vi "Filter Meta.vi"(8 "error in (no error)":errorcluster, 10 "Element In":refnum<class "Config Element.lvclass">, 11 "Overlay Filter in":refnum<class "Overlay Filter.lvclass">) -> (0 "error out":errorcluster, 1 "Filtered Meta":T1[](array[typedef]), 2 "Element":refnum<class "Config Element.lvclass">, 3 "Overlay Filter out":refnum<class "Overlay Filter.lvclass">)   [LabVIEW 2020, in "CDM-Config.lvlib" / "Overlay Filter.lvclass"]
uses:
  Overlay Filter.lvclass
  Config Element/Config Element.lvclass
  Meta Data.ctl
  Overlay Filter.lvclass/Overlay Filter.ctl
  CDM-Config.lvlib
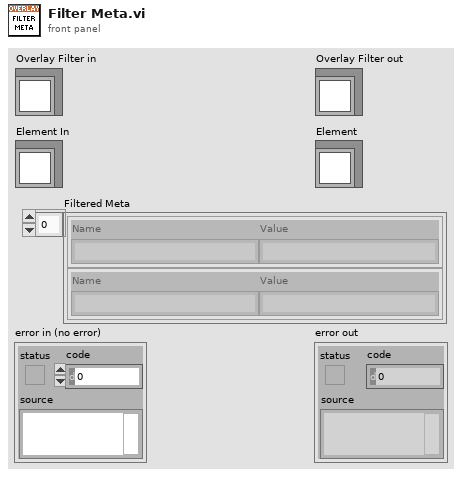
[diagram p1: front panel]
types:
  T1 = typedef "CDM-Config.lvlib/Meta Data.ctl" = cluster{"Name":string, "Value":string}
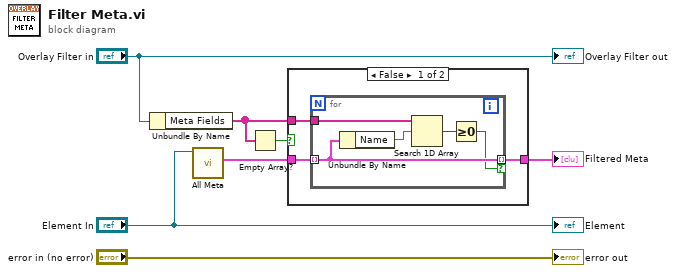
[diagram p0: block diagram]
diagram:
  n1 = Unbundle By Name("Overlay Filter in") -> ("Meta Fields"=w2:string[])
  n2 = call "All Meta.vi"("Config Element In"="Element In") -> ("Meta Data"=w5:T1[])  [unwired: 8 in, 2 out]
  n3 = Empty Array?(array=w2) -> (empty?=w1:bool)
  n4 = case shown="False" w1 {
    tunnel: w5 -> [w10 w16]
    tunnel: [w9 w16] -> w3
    tunnel: w2 -> [w8 _]
    frame False {
      n5 = for {
        tunnel: w8 -> [w15]
        tunnel: w10 -> [w14] mode=indexing
        tunnel: [w14] -> w9 mode=indexing if=w11
        n6 = Unbundle By Name(w14) -> ("Name"=w13:string)
        n7 = Search 1D Array(1D array=w15, element=w13) -> (index of element=w12:i32)  [unwired: 1 in]
        n8 = Greater Or Equal To 0?(x=w12) -> (x >= 0?=w11:bool)
      }
    }
    frame True {
    }
  }
  "Filtered Meta" <- w3
  "error out" <- "error in (no error)"
  "Overlay Filter out" <- "Overlay Filter in"
  "Element" <- "Element In"
